vi "Get Zero Offset Mode.vi"(8 "error in (no error)":errorcluster, 11 "VISA resource name":refnum<visa-resource-name>) -> (0 "error out":errorcluster, 1 "Reference Value":dbl format="%.4f", 2 "Zero Offset Mode":u16, 3 "VISA resource name out":refnum<visa-resource-name>, 4 "Reference Value Units":i32)   [LabVIEW 2014, in "Fluke 5XXX Series Multicalibrators.lvlib"]
doc: "This VI returns the zero offset for the pressure module or capacitance measurement using the oscilloscope option.\n\nNote:\n\nThis VI is available only for instrument models 5500A and 5520A with oscilloscope option SC600 (SC1100) or option 700P (pressure modules)."
uses:
  Fluke 5XXX Series Multicalibrators.lvlib
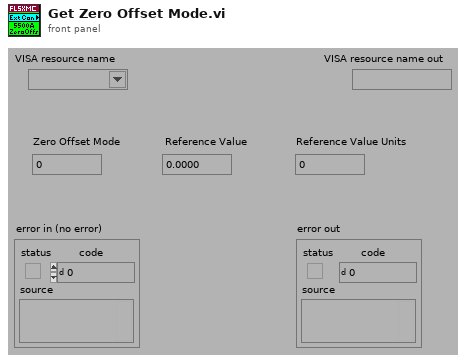
[diagram p1: front panel]
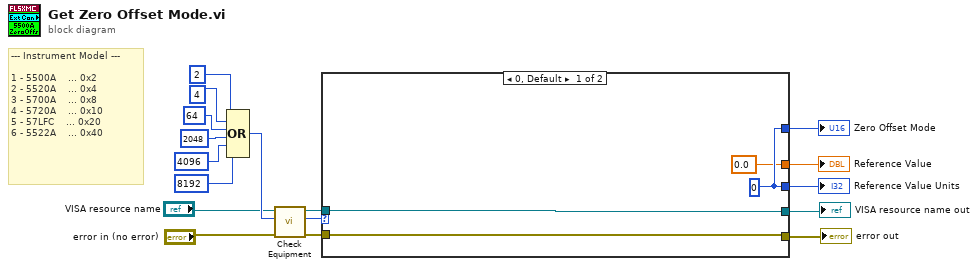
[diagram p0: block diagram]
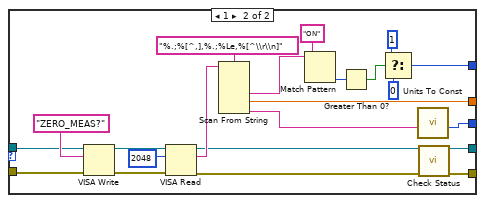
[diagram p2: hidden frame]
diagram:
  # "--- Instrument Model ---\n\n1 - 5500A    ... 0x2\n2 - 5520A    ... 0x4\n3 - 5700A    ... 0x8\n4 - 5720A    ... 0x10\n5 - 57LFC    ... 0x20\n6 - 5522A    ... 0x40"
  n1 = Compound Arithmetic op=OR(2 ("Numeric"), 4 ("Numeric"), 64 ("Numeric"), 2048 ("Numeric"), 4096 ("Numeric"), 8192 ("Numeric")) -> (w9:i32)
  n2 = call "Check Equipment.vi"("error in (no error)"="error in (no error)", "Bit Mask"=w9, "VISA resource name"="VISA resource name") -> ("error out"=w17:errorcluster, "Present?"=w16:u32, "VISA resource name out"=w15:refnum<visa-resource-name>)  [unwired: 6 in]
  n3 = case shown="0, Default" w16 {
    tunnel: [w21 w37] -> w6
    tunnel: [w20 w36] -> w5
    tunnel: w17 -> [w21 w39]
    tunnel: w15 -> [w20 w38]
    tunnel: [w19 w24] -> w4
    tunnel: [w19 w23] -> w2
    tunnel: [0.0 w22] -> w3
    frame 0, Default {
      w19 = 0
    }
    frame 1 {
      n4 = VISA Write(VISA resource name=w38, write buffer="ZERO_MEAS?", error in (no error)=w39) -> (VISA resource name out=w42:refnum<visa-resource-name>, error out=w41:errorcluster)  [unwired: 1 out]
      n5 = VISA Read(VISA resource name=w42, byte count=u32 2048 ("byte count (0)"), error in (no error)=w41) -> (VISA resource name out=w32:refnum<visa-resource-name>, read buffer=w34:string, error out=w33:errorcluster)  [unwired: 1 out]
      n6 = Scan From String(format string="%.;%[^,],%.;%Le,%[^\\r\\n]", input string=w34) -> (output 1=w26:string, output 2=w22:dbl, output 3=w25:string)  [unwired: 5 in, 3 out]
      n7 = Match Pattern(string=w26, regular expression="ON") -> (offset past match=w30:i32)  [unwired: 1 in, 3 out]
      n8 = Greater Than 0?(x=w30) -> (x > 0?=w27:bool)
      n9 = Select(t=u16 1 ("f"), s=w27, f=u16 0) -> (s? t:f=w23:u16)
      n10 = call "Units To Const.vi"("Units"=w25) -> ("Const"=w24:i32)  [unwired: 10 in]
      n11 = call "Check Status.vi"("VISA resource name"=w32, "error in (no error)"=w33) -> ("VISA resource name out"=w36:refnum<visa-resource-name>, "error out"=w37:errorcluster)  [unwired: 12 in]
    }
  }
  "Zero Offset Mode" <- w2
  "Reference Value" <- w3
  "Reference Value Units" <- w4
  "VISA resource name out" <- w5
  "error out" <- w6
